vi "speed_limit_setup.vi"(9 "Down Limit":dbl, 10 "Up Limit":dbl, 11 "Speed":dbl) -> (1 "String out":string, 2 "String out 2":string, 3 "String out 3":string)   [LabVIEW 2017]
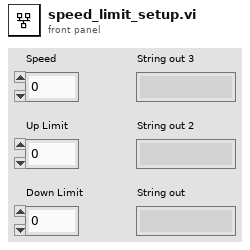
[diagram p1: front panel]
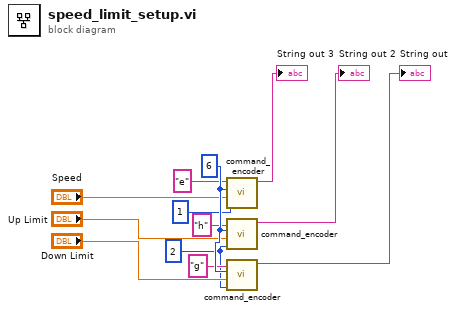
[diagram p0: block diagram]
diagram:
  w12 = 6
  w8 = 2
  n1 = call "command_encoder.vi"("String in"="e", "Numeric"=w12, "Speed"="Speed", "Numeric 2"=1) -> ("String out"=→"String out 3":string)  [unwired: 6 in]
  n2 = call "command_encoder.vi"("String in"="h", "Numeric"=w12, "Speed"="Up Limit", "Numeric 2"=w8) -> ("String out"=→"String out 2":string)  [unwired: 6 in]
  n3 = call "command_encoder.vi"("String in"="g", "Numeric"=w12, "Speed"="Down Limit", "Numeric 2"=w8) -> ("String out"=→"String out":string)  [unwired: 6 in]
